vi "Configure.vi"(8 "error in":errorcluster, 10 "name":string="CRDS", 11 "tCRD in":refnum<class "Aircraft OPCCRD.lvclass">) -> (0 "error out":errorcluster, 3 "tCRD out":refnum<class "Aircraft OPCCRD.lvclass">)   [LabVIEW 2015, in "Aircraft OPCCRD.lvclass"]
doc: "Configures the CRDS for operation and starts all DAQmx tasks associated with the instrument. This VI overrides the parent VI in the Instrument class."
uses:
  Aircraft OPCCRD.lvclass
  Reusable/Instrument/state.ctl
  Reusable/Session APIs/File Access/Config Data/Config Session.ctl
  Reusable/Session APIs/File Access/Config Data/Config Data.lvclass
  Data/tCRD Data.lvclass
  Reusable/Session APIs/File Access/Config Data/Config Data.lvclass/Config Data.ctl
  Reusable/Instrument/Instrument.lvclass/Instrument.ctl
  Reusable/Session APIs/File Access/Config Data/Accessors/Write Cfg Path.vi
  Reusable/Instrument/Write Cfg Session.vi
  Reusable/CRDS/Main/Write Data.vi
  Reusable/CRDS/Main/CRDS.lvclass
  Reusable/Instrument/Instrument.lvclass
  <userlib>/_Session Fwk/Session - Root.lvclass
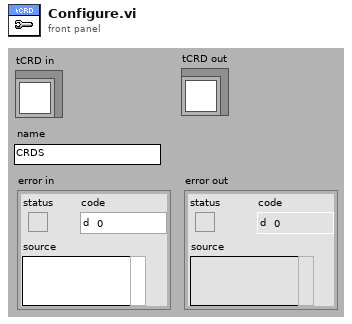
[diagram p1: front panel]
types:
  T1 = typedef "Config Data.lvclass/Config Session.ctl" = refnum<data-value>
  T2 = typedef "Instrument.lvclass/state.ctl" = enum8{"Configure", "Acquire", "Wait", "Quit", "Handle Error", "NOOP"}
  T3 = typedef "Session - Root.lvclass/Session Handle.ctl" = refnum<data-value>
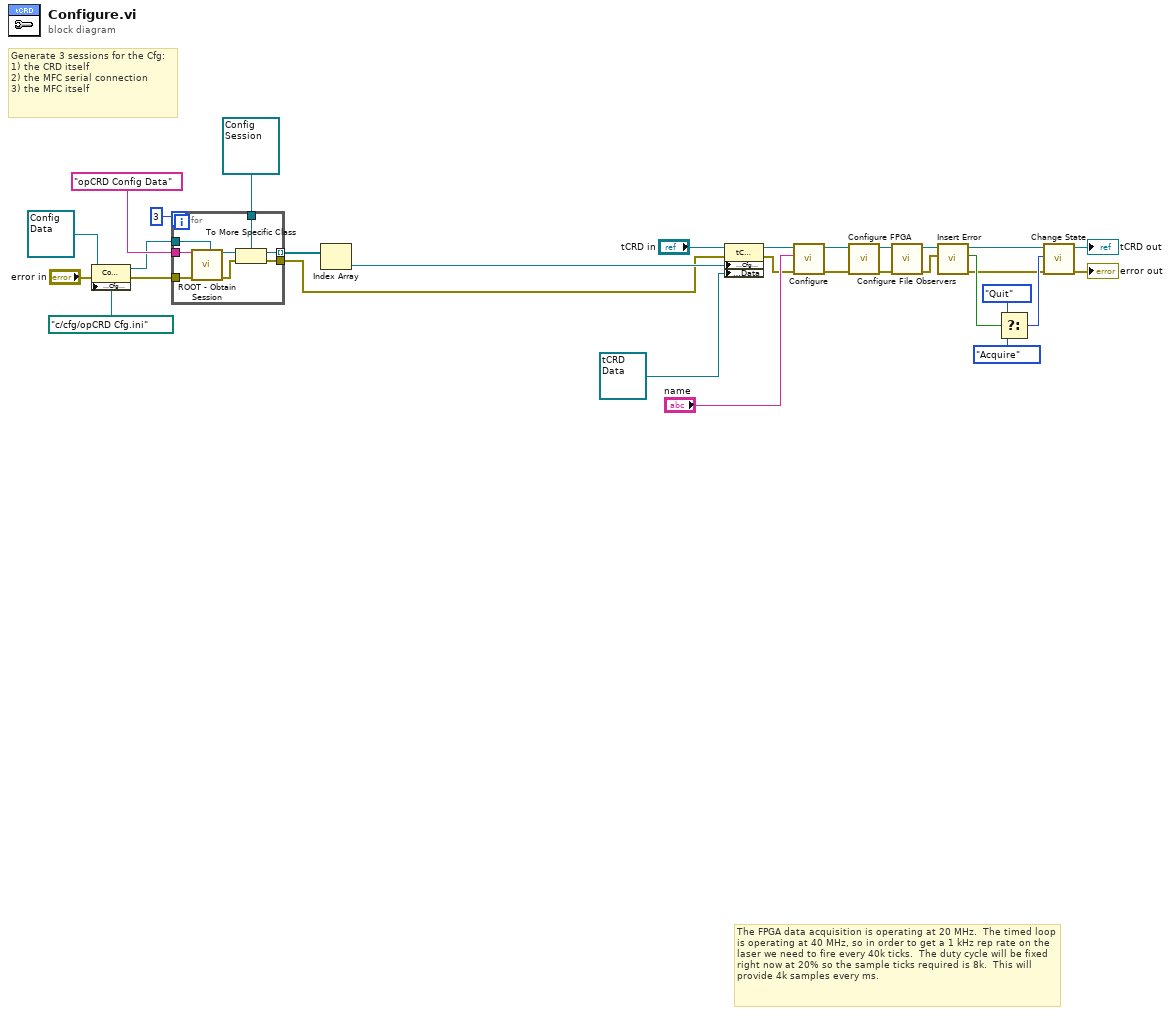
[diagram p0: block diagram]
diagram:
  # "Generate 3 sessions for the Cfg:\n1) the CRD itself\n2) the MFC serial connection\n3) the MFC itself"
  # "The FPGA data acquisition is operating at 20 MHz.  The timed loop is operating at 40 MHz, so in order to get a 1 kHz rep rate on the laser we need to fire every 40k ticks.  The duty cycle will be fixed right now at 20% so the sample ticks required is 8k.  This will provide 4k samples every ms."
  n1 = property class="Config Data"(reference=refnum<class "Config Data.lvclass"> refnum ("Config Data"), error in="error in", "Accessors:Cfg Path"=path "c:/cfg/opCRD Cfg.ini" ("Path")) -> (reference out=w13:refnum<class "Config Data.lvclass">, error out=w14:errorcluster)
  n2 = for {
    N: 3 -> [_]
    tunnel: [w37] -> w21 mode=indexing
    tunnel: "opCRD Config Data" ("Session Name ()") -> [w33]
    tunnel: T1 refnum ("Session Handle") -> [w32]
    tunnel: w14 -> [w35]
    tunnel: [w36] -> w4
    tunnel: w13 -> [w31]
    n3 = call <userlib>:"ROOT - Obtain Session.vi"("Session Name ()"=w33, "OBJ - Session"=w31, "error in (no error)"=w35) -> ("Session Handle"=w38:T3, "error out"=w34:errorcluster)  [unwired: 10 in, 1 out]
    n4 = To More Specific Class(target class=w32, reference=w38, error in=w34) -> (specific class reference=w37:T1, error out=w36:errorcluster)
  }
  n5 = Index Array(array=w21) -> (element=w6:T1)  [unwired: 1 in]
  n6 = property class="tCRD"(reference="tCRD in", error in=w4, "Accessors:Cfg Session"=w6, "Data Access:Data"=refnum<class "tCRD Data.lvclass"> refnum ("tCRD Data")) -> (reference out=w7:refnum<class "Aircraft OPCCRD.lvclass">, error out=w5:errorcluster)
  n7 = call-parent "Configure.vi"("error in"=w5, "name"="name", "CRDS in"=w7) -> ("error out"=w2:errorcluster, "CRDS out"=w3:refnum<class "Aircraft OPCCRD.lvclass">)  [unwired: 7 in]
  n8 = call "Configure FPGA.vi"("error in"=w2, "tCRD in"=w3) -> ("error out"=w11:errorcluster, "tCRD out"=w12:refnum<class "Aircraft OPCCRD.lvclass">)  [unwired: 8 in]
  n9 = call "Configure File Observers.vi"("error in"=w11, "tCRD in"=w12) -> ("error out"=w9:errorcluster, "tCRD out"=w10:refnum<class "Aircraft OPCCRD.lvclass">)  [unwired: 8 in]
  n10 = call "Insert Error.vi"("err"=w9, "Instrument in"=w10) -> ("error out"=w24:errorcluster, "error?"=w27:bool, "Instrument out"=w25:refnum<class "Aircraft OPCCRD.lvclass">)  [unwired: 7 in]
  n11 = Select(t=state."Quit" ("instr state"), s=w27, f=state."Acquire" ("instr state")) -> (s? t:f=w26:T2)
  n12 = call "Change State.vi"("error in"=w24, "instr state"=w26, "Instrument in"=w25) -> ("error out"=→"error out":errorcluster, "Instrument out"=→"tCRD out":refnum<class "Aircraft OPCCRD.lvclass">)  [unwired: 7 in]
